vi "Tool_Unicode Update Graph Chart Labels.vi"(6 "Caption":string, 7 "Interpret as Unicode (T)":bool=TRUE, 8 "error in (no error)":errorcluster, 9 "Y Axis Label":string, 10 "X Axis Label":string, 11 "GrphChrt Ref":refnum<vi>) -> (0 "error out":errorcluster, 3 "GrphChrt Ref":refnum<vi>)   [LabVIEW 2009]
panel:
  # "``"
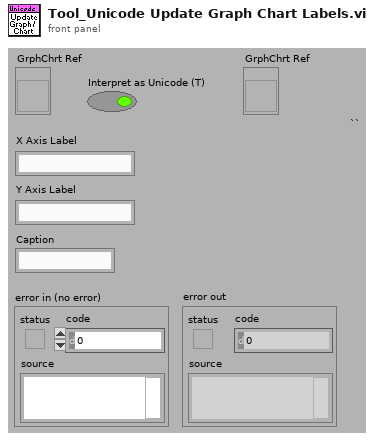
[diagram p1: front panel]
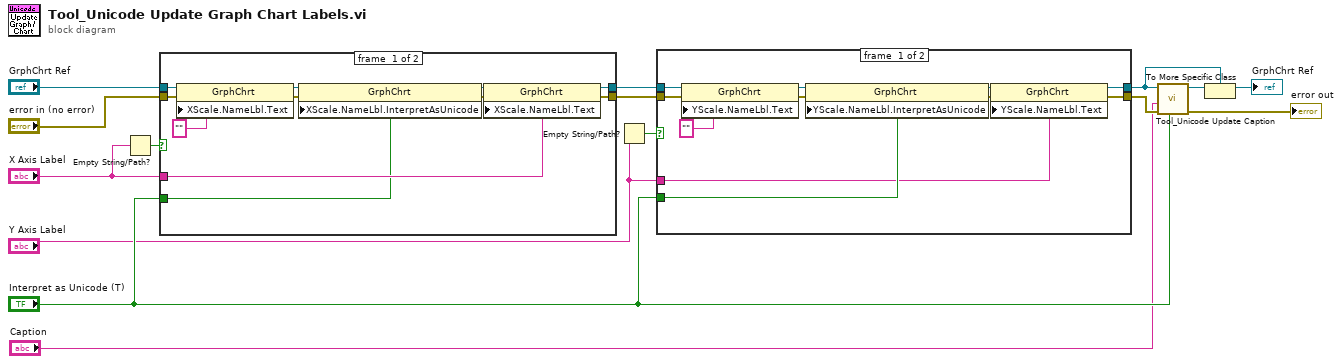
[diagram p0: block diagram]
diagram:
  n1 = Empty String/Path?(string/path="X Axis Label") -> (empty?=w13:bool)
  n2 = case shown="False" w13 {
    tunnel: "X Axis Label" -> [w17 _]
    tunnel: "GrphChrt Ref" -> [w20 w28]
    tunnel: "error in (no error)" -> [w21 w27]
    tunnel: [w18 w28] -> w14
    tunnel: "Interpret as Unicode (T)" -> [w16 _]
    tunnel: [w19 w27] -> w11
    frame #0 {
      n3 = property class="GrphChrt"(reference=w20, error in=w21, "XScale.NameLbl.Text"="" ("Caption.Text")) -> (reference out=w22:refnum<vi>, error out=w23:errorcluster)
      n4 = property class="GrphChrt"(reference=w22, error in=w23, "XScale.NameLbl.InterpretAsUnicode"=w16) -> (reference out=w25:refnum<vi>, error out=w26:errorcluster)
      n5 = property class="GrphChrt"(reference=w25, error in=w26, "XScale.NameLbl.Text"=w17) -> (reference out=w18:refnum<vi>, error out=w19:errorcluster)
    }
    frame #1 {
    }
  }
  n6 = Empty String/Path?(string/path="Y Axis Label") -> (empty?=w12:bool)
  n7 = case shown="False" w12 {
    tunnel: "Y Axis Label" -> [w33 _]
    tunnel: [w29 w41] -> w10
    tunnel: w11 -> [w32 w41]
    tunnel: w14 -> [w31 w40]
    tunnel: "Interpret as Unicode (T)" -> [w34 _]
    tunnel: [w30 w40] -> w7
    frame #0 {
      n8 = property class="GrphChrt"(reference=w31, error in=w32, "YScale.NameLbl.Text"="" ("Caption.Text")) -> (reference out=w35:refnum<vi>, error out=w36:errorcluster)
      n9 = property class="GrphChrt"(reference=w35, error in=w36, "YScale.NameLbl.InterpretAsUnicode"=w34) -> (reference out=w38:refnum<vi>, error out=w39:errorcluster)
      n10 = property class="GrphChrt"(reference=w38, error in=w39, "YScale.NameLbl.Text"=w33) -> (reference out=w30:refnum<vi>, error out=w29:errorcluster)
    }
    frame #1 {
    }
  }
  n11 = call "Tool_Unicode Update Caption.vi"("Interpret as Unicode (T)"="Interpret as Unicode (T)", "error in (no error)"=w10, "Caption"="Caption", "Control Reference"=w7) -> ("error out"=→"error out":errorcluster, "Control Reference"=w8:refnum<vi>)  [unwired: 4 in]
  n12 = To More Specific Class(target class=w7, reference=w8) -> (specific class reference=→"GrphChrt Ref":refnum<vi>)  [unwired: 1 in, 1 out]
